vi "Preset START WAIT Time.vi"(8 "error in (no error)":errorcluster, 10 "Time":dbl min=0.0 max=99.9 step=0.1 format="%.1f", 11 "VISA resource in":refnum<visa-resource-name>) -> (0 "error out":errorcluster, 3 "VISA resource out":refnum<visa-resource-name>)   [LabVIEW 2025, in "Chroma 19572.lvlib"]
doc: "This VI writes to the instrument the AUTO RANGE state."
uses:
  <instrlib>/Chroma 19572/Chroma 19572.lvlib
panel:
  # "0 = OFF\n0,1 to 99,9 sec"
  # "PreSet START WAIT time befor GB test"
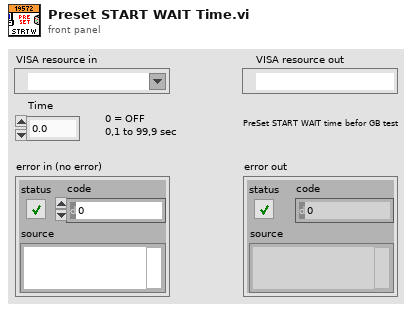
[diagram p1: front panel]
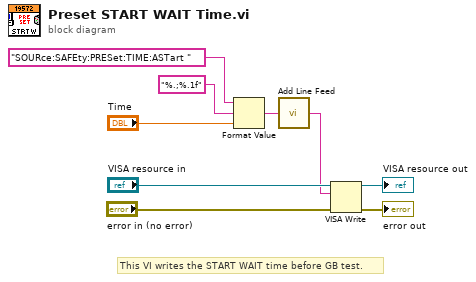
[diagram p0: block diagram]
diagram:
  # "This VI writes the START WAIT time before GB test."
  n1 = Format Value(string ("")="SOURce:SAFEty:PRESet:TIME:ASTart ", format string="%.;%.1f", value (0)="Time") -> (output string=w2:string)
  n2 = call <instrlib>:"Add Line Feed.vi"("Command string"=w2) -> ("Concatenated string"=w1:string)  [unwired: 4 in]
  n3 = VISA Write(VISA resource name="VISA resource in", write buffer=w1, error in (no error)="error in (no error)") -> (VISA resource name out=→"VISA resource out":refnum<visa-resource-name>, error out=→"error out":errorcluster)  [unwired: 1 out]
